vi "runsample(playground_module).vi"() -> ()   [LabVIEW 2010]
panel:
  out "VISA resource out 3":refnum<visa-resource-name>="ASRL2::INSTR"
  in  "VISA resource name 3":refnum<visa-resource-name>="ASRL2::INSTR"
  in  "error in 3":errorcluster
  out "error out 3":errorcluster
  out "VISA resource out 2":refnum<visa-resource-name>="ASRL2::INSTR"
  in  "VISA resource name 2":refnum<visa-resource-name>="ASRL2::INSTR"
  in  "error in 2":errorcluster
  out "error out 2":errorcluster
  out "VISA resource out":refnum<visa-resource-name>="ASRL2::INSTR"
  in  "VISA resource name":refnum<visa-resource-name>="ASRL2::INSTR"
  in  "error in":errorcluster
  out "error out":errorcluster
  in  "Start Run":bool
  in  "DataFile":path
  in  "stop":bool
  in  "Number of Repeats":i32=1
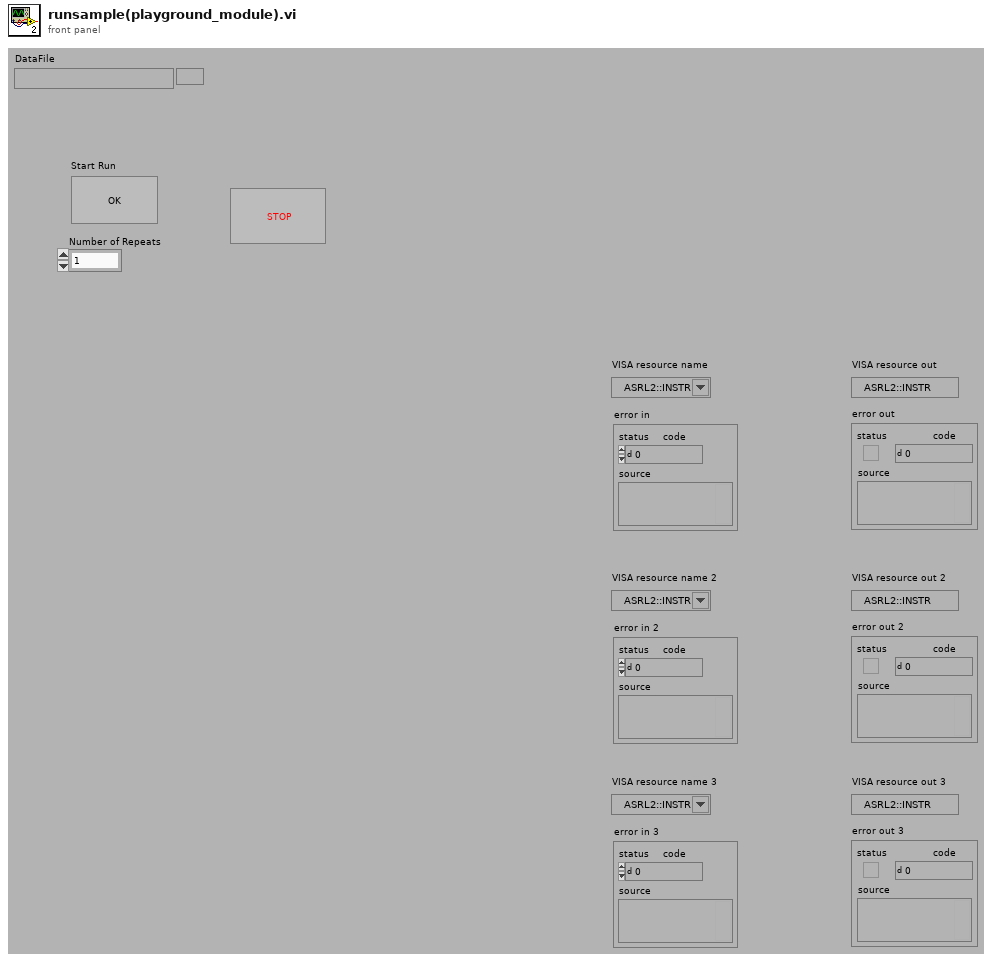
[diagram p1: front panel]
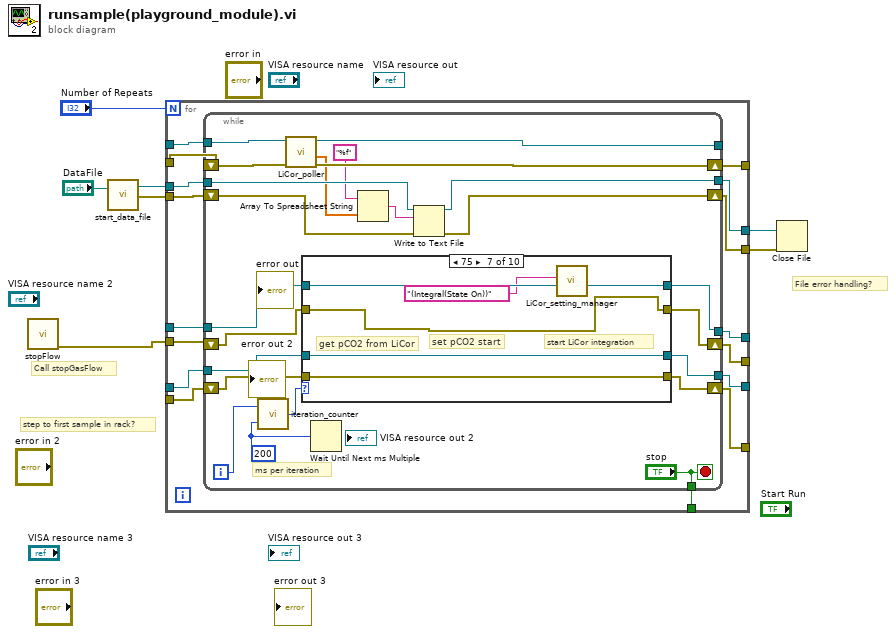
[diagram p0: block diagram]
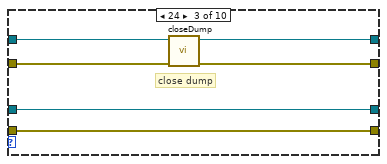
[diagram p4: hidden frame]
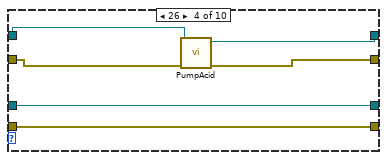
[diagram p5: hidden frame]
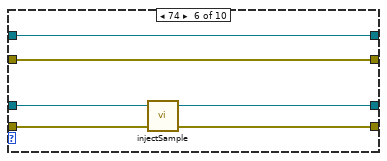
[diagram p7: hidden frame]
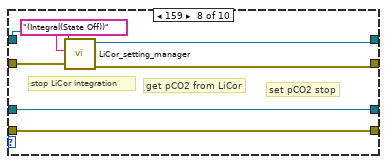
[diagram p8: hidden frame]
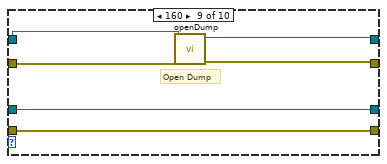
[diagram p9: hidden frame]
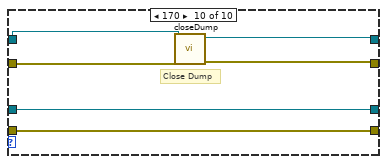
[diagram p10: hidden frame]
diagram:
  # "File error handling?"
  # "Call stopGasFlow"
  # "step to first sample in rack?"
  n1 = call "stopFlow.vi"() -> ("error out"=w14:errorcluster)  [unwired: 10 in, 1 out]
  n2 = call "start_data_file.vi"("DataFile"="DataFile") -> ("error out"=w2:errorcluster, "Byte Stream File Refnum"=w1:refnum<file>)  [unwired: 9 in]
  n3 = for {
    N: "Number of Repeats" -> [_]
    tunnel: [w34] -> w17
    tunnel: [w33] -> w16
    tunnel: w1 -> [w32]
    tunnel: [w30] -> w15
    tunnel: w14 -> [w31]
    tunnel: w2 -> [w29]
    tunnel: [w28] -> w13
    tunnel: [w27] -> w12
    tunnel: [w26] -> w11
    tunnel: [w25] -> w10
    tunnel: [w24] -> w9
    tunnel: [w23] -> w8
    tunnel: [w22] -> w7
    tunnel: [w21] -> w6
    tunnel: [w20] -> w5
    tunnel: [w19] -> w4
    n4 = while {
      tunnel: [w57] -> _
      tunnel: w34 -> [w56]
      shift-right: [w54] -> w23
      shift-left: w33 -> [w55]
      tunnel: w32 -> [w53]
      tunnel: w30 -> [w46]
      tunnel: [w49] -> w28
      shift-right: [w48] -> w27
      shift-left: w29 -> [w52]
      tunnel: ["stop"] -> w26
      tunnel: w25 -> [w44]
      shift-right: [w42] -> w19
      shift-left: w24 -> [w43]
      tunnel: [w41] -> w20
      tunnel: [w40] -> w22
      shift-right: [w39] -> w21
      shift-left: w31 -> [w45]
      i -> [w37]
      stop <- "stop" stop-if-true
      w36 = 200 ("ms between samples")
      # "ms per iteration"
      n5 = call "iteration_counter.vi"("ms per iteration"=w36, "index"=w37) -> ("seconds"=w38:i32)
      n6 = call "LiCor_poller.vi"("error in"=w55, "VISA session in"=w56) -> ("error out"=w54:errorcluster, "data array"=w51:dbl[], "VISA session out"=w57:refnum<visa-resource-name>)  [unwired: 5 in, 2 out]
      n7 = case shown="75" w38 {
        tunnel: w46 -> [w59 w63 w69 w75 w81 w87 w90 w96 w103 w109]
        tunnel: w45 -> [w58 w62 w67 w74 w80 w86 w89 w93 w102 w108]
        tunnel: w44 -> [w61 w65 w70 w77 w79 w85 w92 w99 w105 w111]
        tunnel: w43 -> [w60 w64 w71 w76 w78 w84 w91 w98 w104 w110]
        tunnel: [w60 w64 w71 w76 w78 w82 w91 w98 w104 w110] -> w42
        tunnel: [w61 w65 w70 w77 w79 w83 w92 w99 w105 w111] -> w41
        tunnel: [w59 w63 w68 w73 w81 w87 w90 w95 w100 w106] -> w40
        tunnel: [w58 w62 w66 w72 w80 w86 w89 w94 w101 w107] -> w39
        frame 0, Default {
        }
        frame 1 {
          # "Run Rinse_GetSample"
        }
        frame 24 {
          # "close dump"
          n8 = call "closeDump.vi"("error in"=w67, "VISA resource name"=w69) -> ("error out"=w66:errorcluster, "VISA resource out"=w68:refnum<visa-resource-name>)  [unwired: 8 in]
        }
        frame 26 {
          n9 = call "PumpAcid.vi"("error in"=w74, "VISA resource name"=w75) -> ("error out"=w72:errorcluster, "VISA resource out"=w73:refnum<visa-resource-name>)  [unwired: 8 in]
        }
        frame 60 {
          # "normal flow"
        }
        frame 74 {
          n10 = call "injectSample.vi"("error in"=w84, "VISA resource in"=w85) -> ("error out"=w82:errorcluster, "VISA resource out"=w83:refnum<visa-resource-name>)  [unwired: 2 in]
        }
        frame 75 {
          # "start LiCor integration"
          # "set pCO2 start"
          # "get pCO2 from LiCor"
          n11 = call "LiCor_setting_manager.vi"("string to write"="(Integral(State On))") -> ()  [unwired: 9 in, 2 out]
        }
        frame 159 {
          # "set pCO2 stop"
          # "get pCO2 from LiCor"
          # "stop LiCor integration"
          n12 = call "LiCor_setting_manager.vi"("error in"=w93, "string to write"="(Integral(State Off))", "VISA session in"=w96) -> ("error out"=w94:errorcluster, "VISA session out"=w95:refnum<visa-resource-name>)  [unwired: 7 in]
        }
        frame 160 {
          # "Open Dump"
          n13 = call "openDump.vi"("error in"=w102, "VISA resource name"=w103) -> ("error out"=w101:errorcluster, "VISA resource out"=w100:refnum<visa-resource-name>)  [unwired: 8 in]
        }
        frame 170 {
          # "Close Dump"
          n14 = call "closeDump.vi"("error in"=w108, "VISA resource name"=w109) -> ("error out"=w107:errorcluster, "VISA resource out"=w106:refnum<visa-resource-name>)  [unwired: 8 in]
        }
      }
      n15 = Wait Until Next ms Multiple(millisecond multiple=w36) -> ()  [unwired: 1 out]
      n16 = Array To Spreadsheet String(array=w51, 3:"%f") -> (spreadsheet string=w50:string)  [unwired: 1 in]
      n17 = Write to Text File(file (use dialog)=w53, text=w50, error in=w52) -> (refnum out=w49:refnum<file>, error out=w48:errorcluster)  [unwired: 1 in, 1 out]
    }
  }
  n18 = Close File(refnum=w13, error in=w12) -> ()  [unwired: 2 out]
